vi "MOKE_meas.vi"() -> ()   [LabVIEW 2017]
doc: "Use this template to build a producer/consumer design pattern with events to produce queue items. Use this design pattern instead of the User Interface Event Handler pattern for user interfaces when you want to execute code asynchronously in response to an event without slowing the user interface responsiveness."
uses:
  StateMachine.ctl
  Xaxis.ctl
  Yaxis.ctl
  Meas_arrays.ctl
  <vilib>/DAQmx/write.llb/DAQmx Write (Analog DBL 1Chan 1Samp).vi
  <vilib>/DAQmx/read.llb/DAQmx Read (Analog DBL 1Chan 1Samp).vi
  <vilib>/Analysis/baseanly.llb/Mean (DBL).vi
  <vilib>/DAQmx/read.llb/DAQmx Read (Analog 1D DBL 1Chan NSamp).vi
  <vilib>/DAQmx/read.llb/DAQmx Read (Analog 1D Wfm NChan NSamp).vi
  <vilib>/DAQmx/create/channels.llb/DAQmx Create Channel (AO-Voltage-Basic).vi
  <vilib>/DAQmx/miscellaneous.llb/DAQmx Fill In Error Info.vi
  <vilib>/DAQmx/create/channels.llb/DAQmx Create Channel (AI-Voltage-Basic).vi
  <vilib>/express/express shared/transition.llb/Dynamic To Waveform Array.vi
  <vilib>/express/express arith-compare/Formula/Block/exnFormulaBlock how many pts in the wave.vi
  <vilib>/express/express shared/ex_Modify Signal Name.vi
  <vilib>/express/express shared/transition.llb/Waveform Array To Dynamic.vi
  <vilib>/DAQmx/configure/timing.llb/DAQmx Timing (Sample Clock).vi
  <vilib>/express/express arith-compare/Formula/XNode/ExpressFormulaBlockNode.xnode
  <vilib>/Analysis/NI_AALBase.lvlib
  <vilib>/Analysis/NI_AALPro.lvlib
panel:
  out "Magnetic Bgr":dbl format="%0.2f"
  in  "Plot?":bool=TRUE
  in  "Set Field":bool
  in  "Solenoid Current (A)":dbl
  in  "Magnetization Curve":bool
  in  "Averaging":i32
  in  "Next pt (ms)":u32
  in  "Dwell Time (ms)":u32
  in  "stop 2":bool
  in  "Calibration  (V/deg)":dbl=1.0
  in  "DC normalized?":bool
  out "Array":dbl[](array[numeric])
  out "subarray":dbl[](array[numeric])
  out "LockIn A":dbl[][](array[numeric])
  in  "Current Step (A)":dbl
  in  "Up/dn":bool=TRUE
  in  "Actual Current (A)":dbl
  in  "Max Current (A)":dbl
  in  "Min Current (A)":dbl
  in  "Sweep Field":bool
  in  "Enqueue Element":bool
  in  "Magnet position (mm)":dbl
  in  "Magnet Offset (mm)":dbl=12.5
  in  "Reset":bool
  in  "Continuous":bool
  in  "Polarity":bool
  in  "milliseconds to wait":u32=200
  in  "Tab Control":T1(tab)
  out "Temperature (K)":dbl
  in  "New File":bool
  in  "Measurement File":string
  in  "X axis":T2
  in  "Y axis":T3
  out "Lock-in X, Y":T4(graph)
  in  "X axis 3":T2
  out "MOKE 2":T5(graph)
  in  "Save Data":bool
  out "Magnetic Field (mT)":dbl
  in  "X axis 2":T2
  in  "Y axis 2":T3
  out "dm/dH":T5(graph)
  in  "Delete Calibration":bool
  in  "Measure":bool
  in  "Analyzer angle":dbl step=0.2
  out "MOKE Calibration":cluster{dbl[], "Best Linear Fit":dbl[]}[](graph)
  out "Waveform Graph 2":waveform(dbl)[](graph)
  out "Waveform Graph":waveform(dbl)[](graph)
  in  "DAQ Max voltage":dbl=5.0 format="%0.2f"
  in  "DAQ Min voltage":dbl=-5.0 format="%0.2f"
  in  "DAQ Sample Rate (Hz)":dbl=1000.0
  in  "physical channels":tag="Dev1/ai0:1"
  in  "samples per channel":i32=1000
  in  "Lakeshore VISA":refnum<visa-resource-name>="GPIB0::12::INSTR"
  in  "Keithley or myDAQ":bool=TRUE
  in  "Keithley VISA":refnum<visa-resource-name>="GPIB0::20::INSTR"
  in  "myDAQ":bool
  in  "PT1000 Measure":tag="Dev1/ai1:2"
  in  "minimum value Pt":dbl format="%0.2f"
  in  "maximum value Pt":dbl=5.0 format="%0.2f"
  in  "Dc Intensity PT1000":tag="Dev1/ao1"
  in  "Hall-sensor calibration (mV/mT)":dbl=14.0 format="%0.2f"
  in  "maximum value Hall":dbl=5.0 format="%0.2f"
  in  "minimum value Hall":dbl format="%0.2f"
  in  "Dc Intensity Hall":tag="Dev1/ao0"
  in  "Lockin A, Harmonic":bool=TRUE
  in  "LockIn A VISA":refnum<visa-resource-name>="GPIB0::9::INSTR"
  in  "LockIn B VISA":refnum<visa-resource-name>="GPIB0::9::INSTR"
  in  "Lockin B, Harmonic":bool=TRUE
  in  "Dual Lockin":bool
  in  "Detektor DAQ?":bool
  in  "Hall Measure F":tag="Dev1/ai0"
  in  "Hall Measure":tag="Dev1/ai0"
  in  "Detector signal":tag="Dev1/ai3"
  out "PID signal":dbl
  in  "Goal Temperature (K)":dbl=300.0
  in  "Parameters":cluster{"P":dbl, "I":dbl, "D":dbl}={"P"=1.0, "I"=2.0, "D"=0.0}
  in  "PID On/Off":bool
  in  "Plus Resistance":dbl
  in  "Measurement Arrays":T6
  out "Actual Measurement":T7={"Elapsed Time (s)"=0.0, "Hall-Sensor (mT)"=0.0, "LockIn A"=[1.33515e-05, 1.14442e-05, 1.90736e-05, 41.634], "LockIn B"=[1.33515e-05, 1.14442e-05, 1.90736e-05, 41.634], "Dc Intensity (V)"=0.0, "Temperature (K)"=0.0}
  out "StateMachine":T8
  in  "stop":bool
  # "+"
  # "-"
  # "1f"
  # "2f"
  # "1f"
  # "2f"
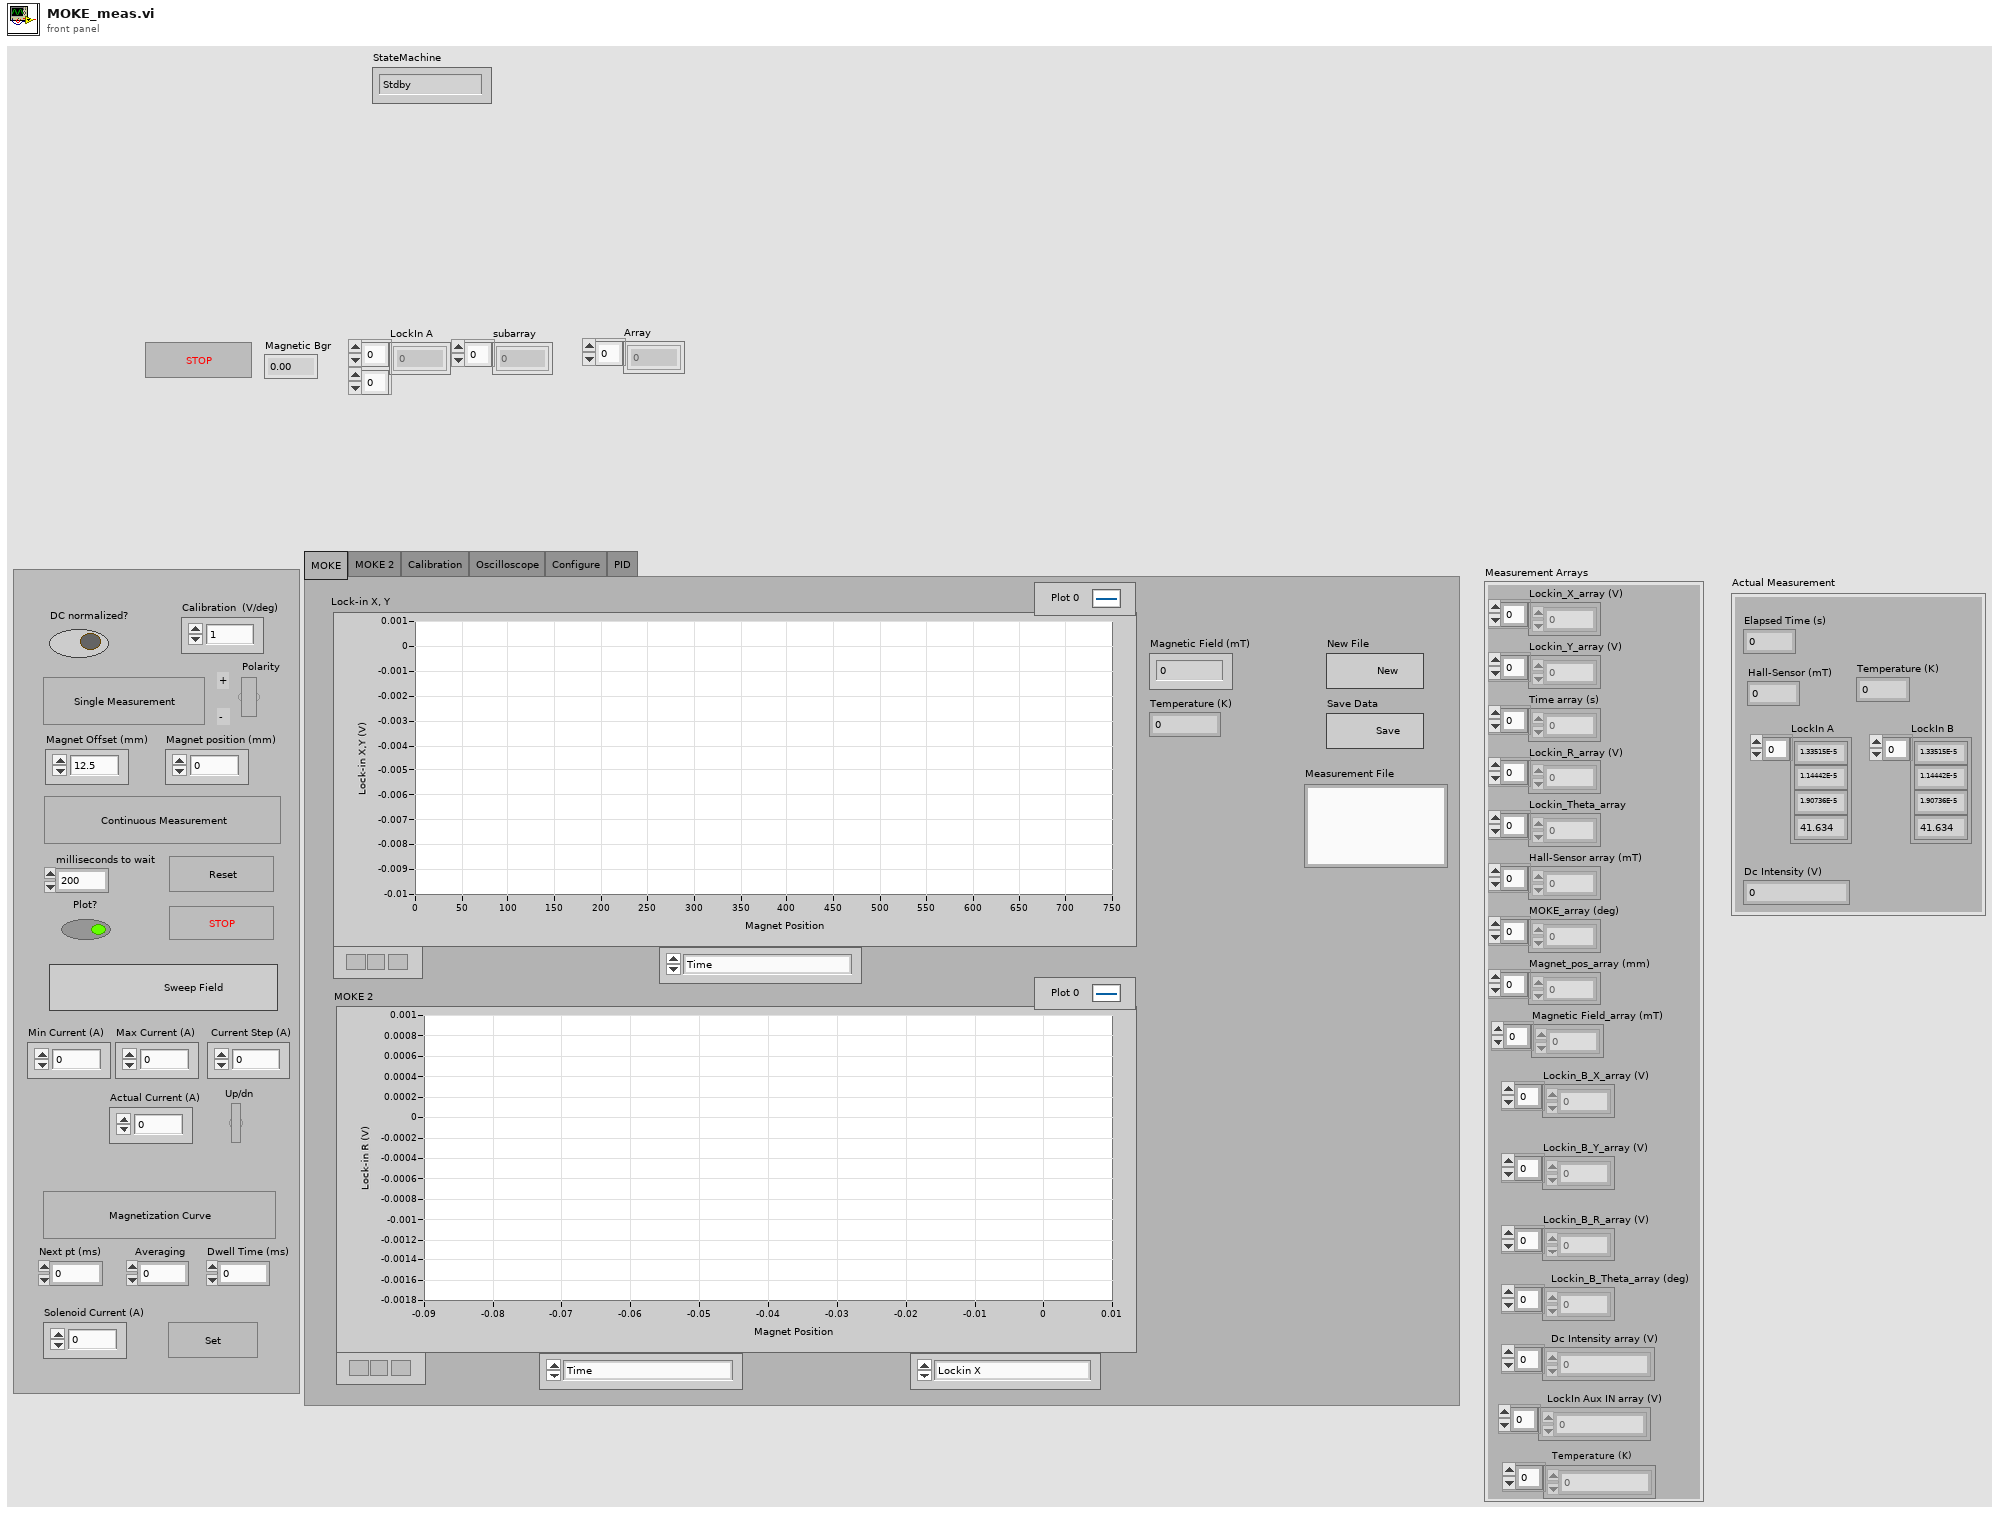
[diagram p1: front panel]
types:
  T1 = enum32{"MOKE", "MOKE 2", "Calibration", "Oscilloscope", "Configure", "PID"}
  T2 = typedef "Xaxis.ctl" = enum16{"Time", "Magnetic Field", "Magnet Position", "Hall Sensor"}
  T3 = typedef "Yaxis.ctl" = enum16{"Lockin X", "Lockin Y", "Lockin R", "Lockin Theta", "MOKE (deg)", "Dc Intensity (V)"}
  T4 = cluster{"Hall-voltage array (V)":dbl[], "Lockin_Y_array (V)":dbl[]}[]
  T5 = cluster{"Magnet_pos_array (mm)":dbl[], "Dc_Voltage_array (V)":dbl[]}
  T6 = typedef "Meas_arrays.ctl" = cluster{"Lockin_X_array (V)":dbl[], "Lockin_Y_array (V)":dbl[], "Time array (s)":dbl[], "Lockin_R_array (V)":dbl[], "Lockin_Theta_array":dbl[], "Hall-Sensor array (mT)":dbl[], "MOKE_array (deg)":dbl[], "Magnet_pos_array (mm)":dbl[], "Magnetic Field_array (mT)":dbl[], "Lockin_B_X_array (V)":dbl[], "Lockin_B_Y_array (V)":dbl[], "Lockin_B_R_array (V)":dbl[], "Lockin_B_Theta_array (deg)":dbl[], "Dc Intensity array (V)":dbl[], "LockIn Aux IN array (V)":dbl[], "Temperature (K)":dbl[]}
  T7 = cluster{"Elapsed Time (s)":dbl, "Hall-Sensor (mT)":dbl, "LockIn A":dbl[], "LockIn B":dbl[], "Dc Intensity (V)":dbl, "Temperature (K)":dbl}
  T8 = typedef "StateMachine.ctl" = enum16{"Stdby", "Configure", "Acquire", "Continuous", "Oscilloscope", "Magnetization", "Calibrate", "PID"}
  T9 = cluster{"Elapsed Time (s)":dbl, "Hall-sensor (mT)":dbl, "LockIn A":dbl[], "LockIn B":dbl[], "Dc Intensity (V)":dbl, "Temperature (K)":dbl}
  T10 = cluster{"Hall-voltage array (V)":dbl[], "Dc Intensity array (V)":dbl[]}
  T11 = cluster{"Hall-voltage array (V)":dbl[], "MOKE_array (deg)":dbl[]}
  T12 = enum16{"open", "replace", "create", "open or create", "replace or create", "replace or create with confirmation"}
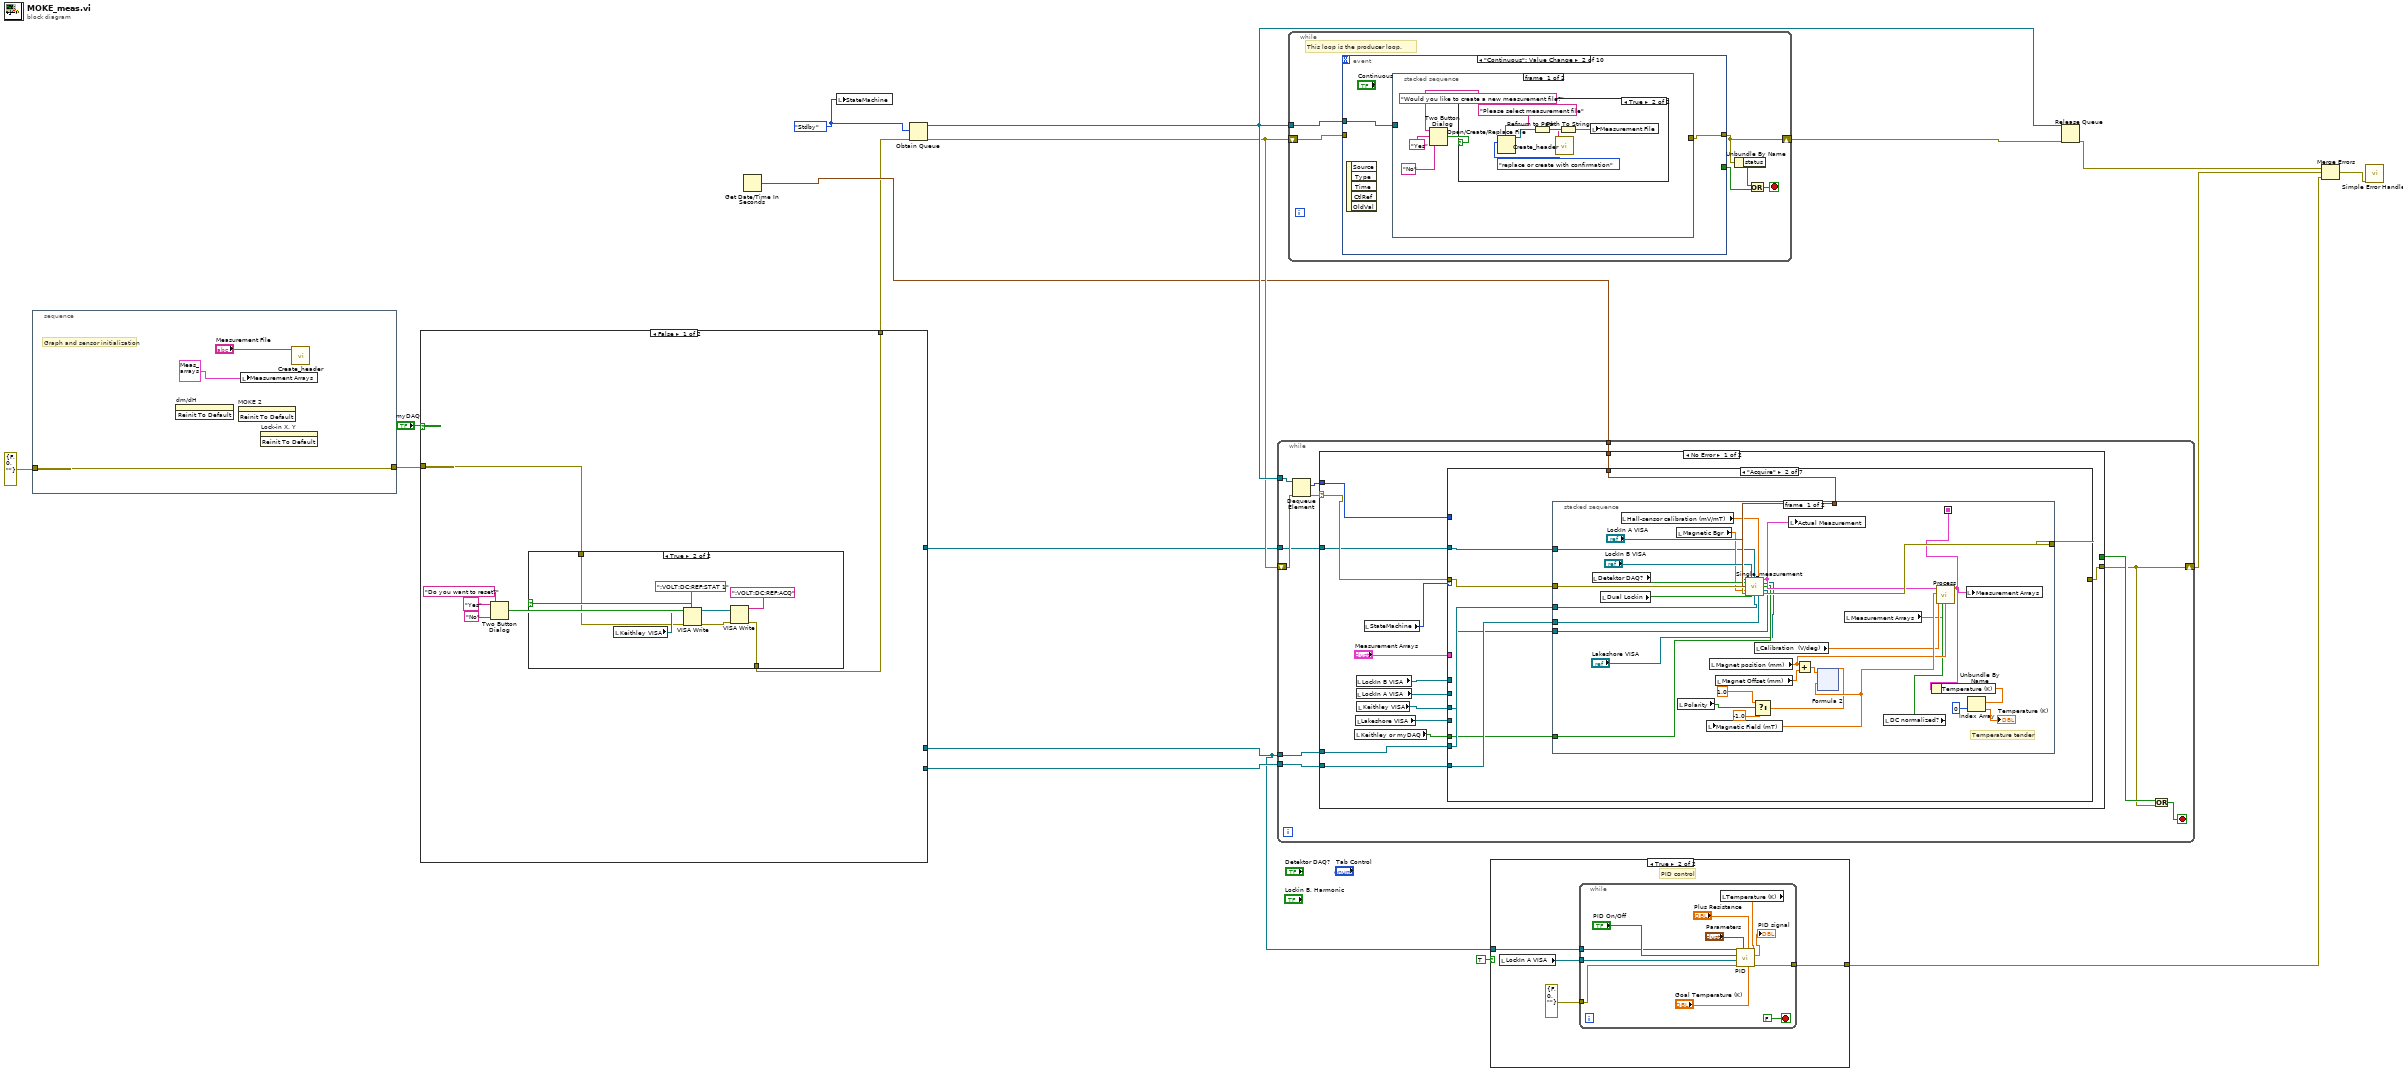
[diagram p0: block diagram]
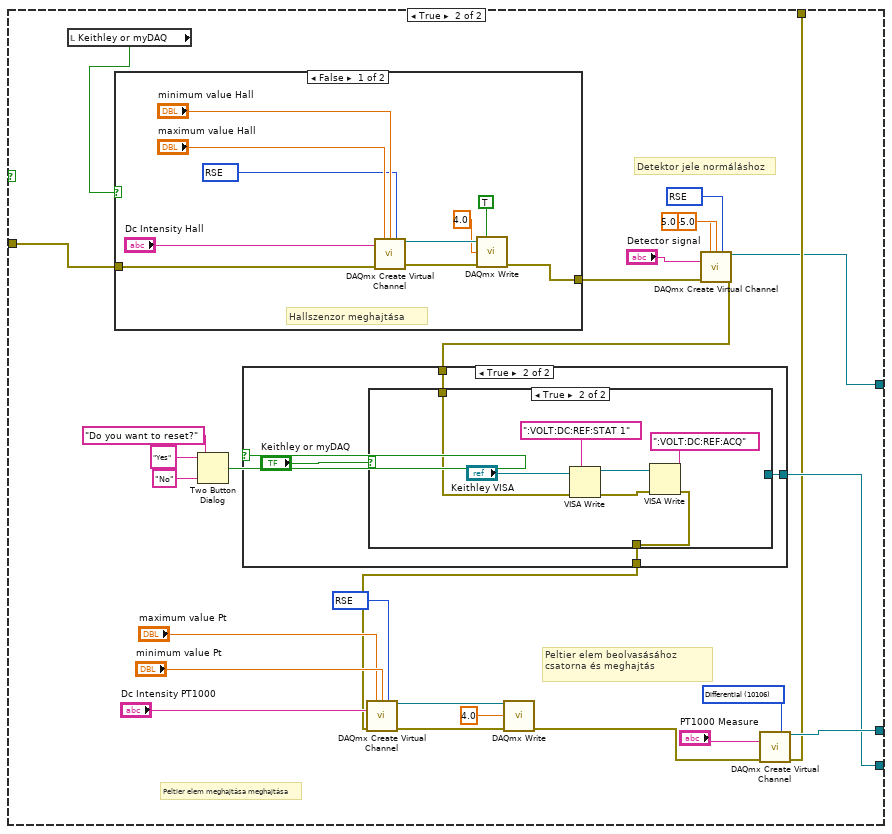
[diagram p4: hidden frame]
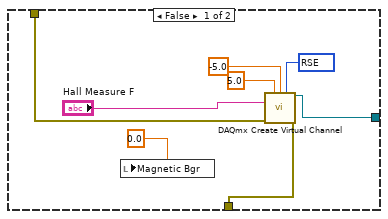
[diagram p6: hidden frame]
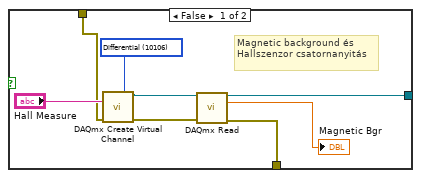
[diagram p7: hidden frame]
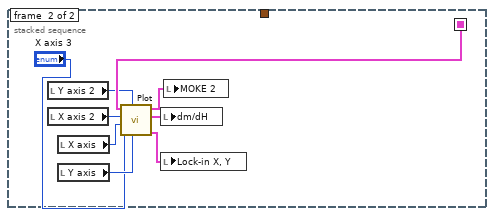
[diagram p9: hidden frame]
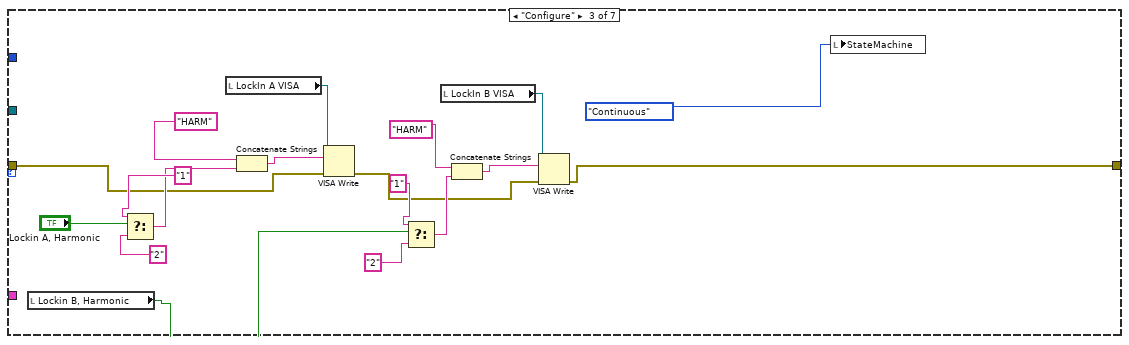
[diagram p10: hidden frame]
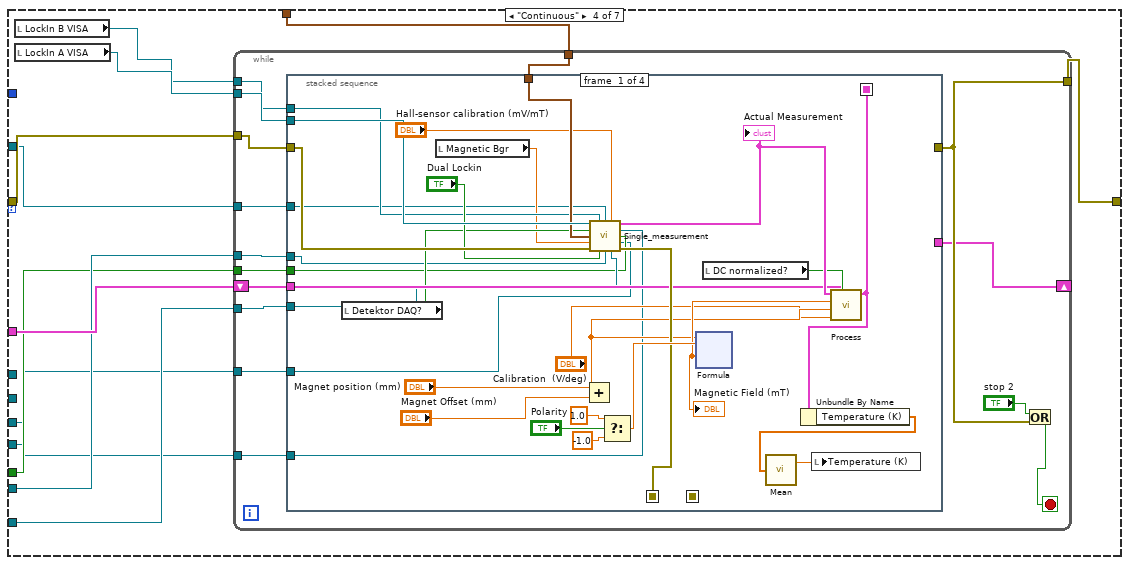
[diagram p11: hidden frame]
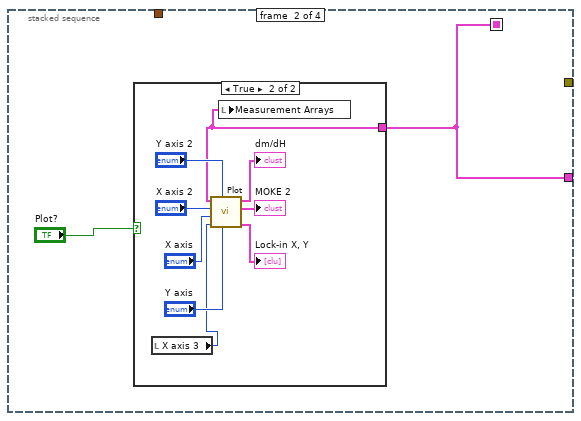
[diagram p12: hidden frame]
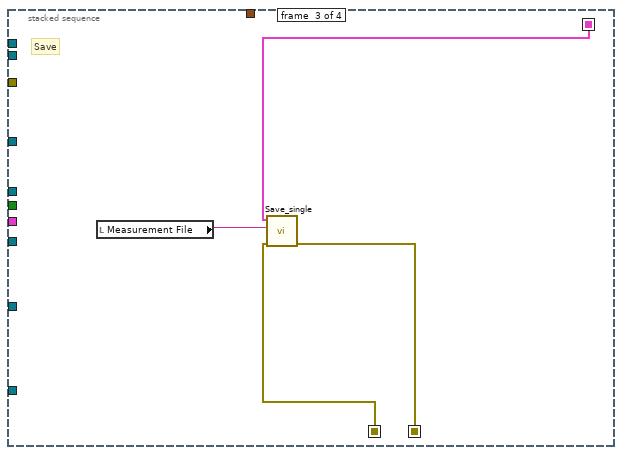
[diagram p14: hidden frame]
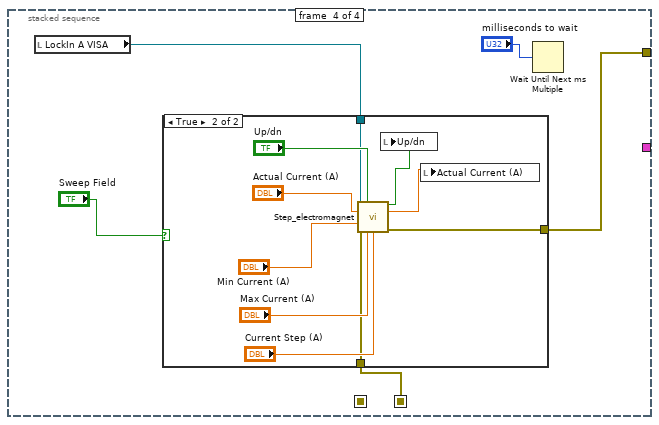
[diagram p15: hidden frame]
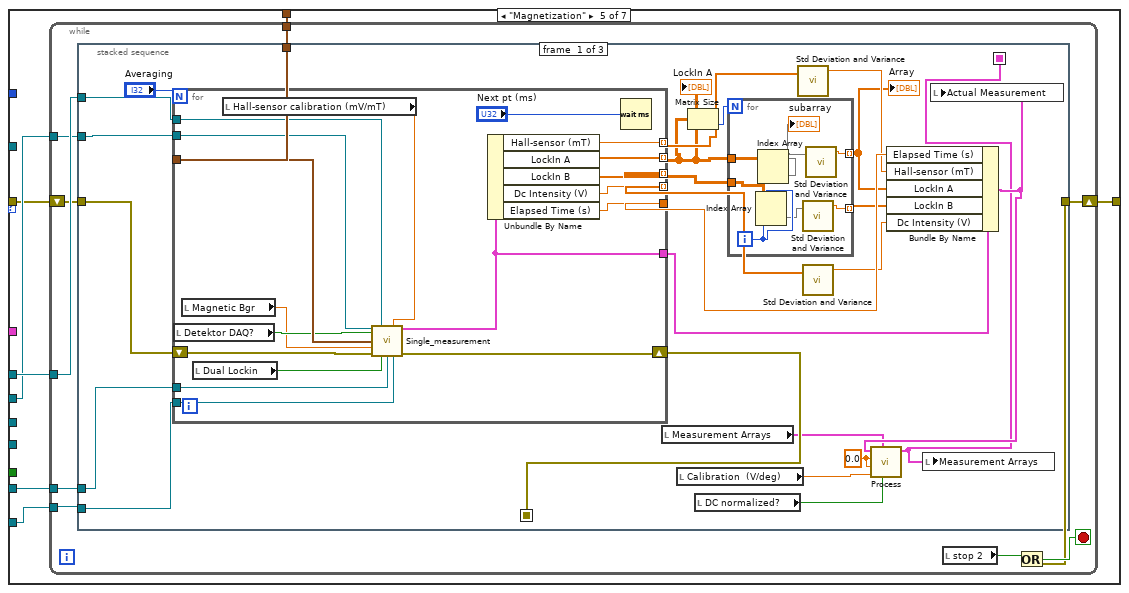
[diagram p17: hidden frame]
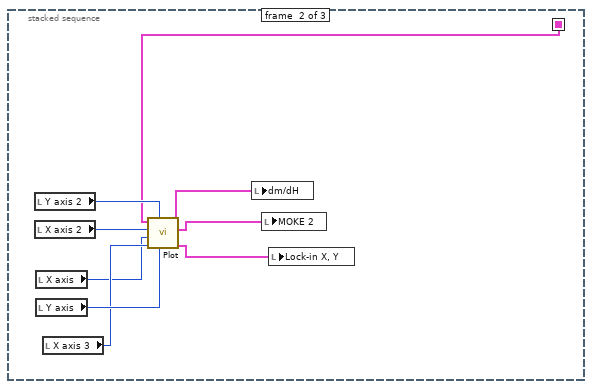
[diagram p18: hidden frame]
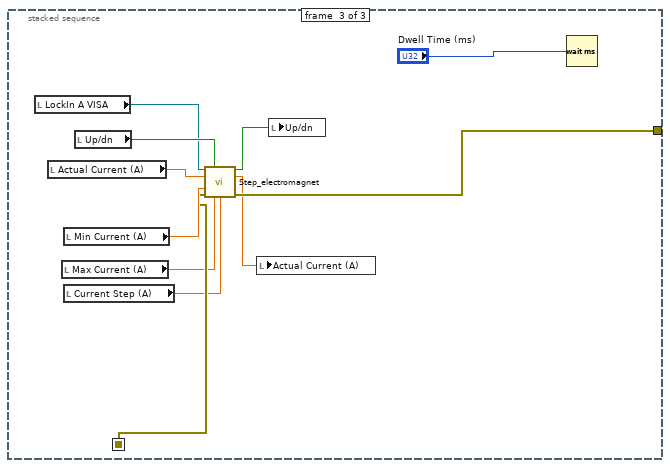
[diagram p19: hidden frame]
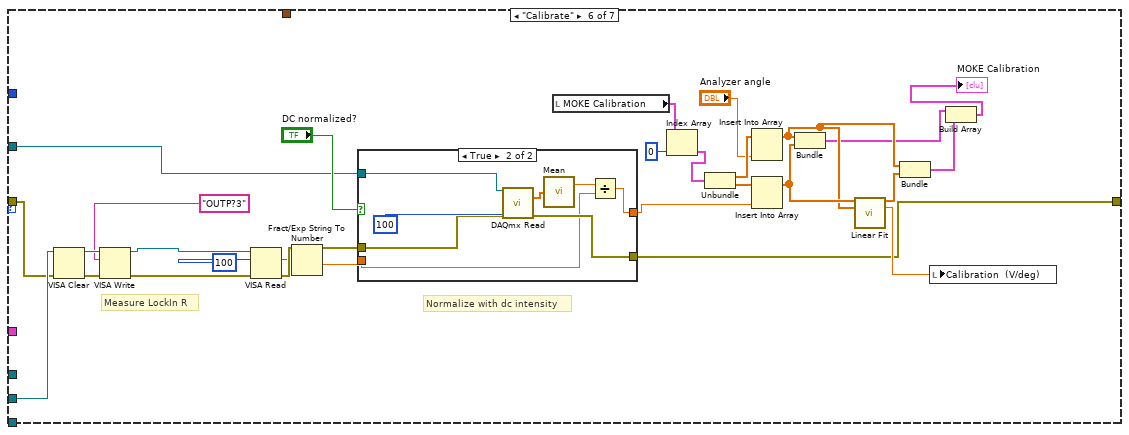
[diagram p20: hidden frame]
diagram:
  w13 = StateMachine."Stdby" ("Enum")
  n1 = stacked-sequence {
    tunnel: errorcluster {"status"=FALSE, "code"=0, "source"=""} ("error out") -> [w20]
    tunnel: [w20] -> w8
    frame #0 {
      # "Graph and sensor initialization"
      n2 = invoke on="dm/dH" class="XYGraph (strict)" method="Reinit To Default"() -> ()  [unwired: 3 in, 3 out]
      n3 = invoke on="MOKE 2" class="XYGraph (strict)" method="Reinit To Default"() -> ()  [unwired: 3 in, 3 out]
      n4 = local write "Measurement Arrays"(T6 {"Lockin_X_array (V)"=[], "Lockin_Y_array (V)"=[], "Time array (s)"=[], "Lockin_R_array (V)"=[], "Lockin_Theta_array"=[], "Hall-Sensor array (mT)"=[], "MOKE_array (deg)"=[], "Magnet_pos_array (mm)"=[], "Magnetic Field_array (mT)"=[], "Lockin_B_X_array (V)"=[], "Lockin_B_Y_array (V)"=[], "Lockin_B_R_array (V)"=[], "Lockin_B_Theta_array (deg)"=[], "Dc Intensity array (V)"=[], "LockIn Aux IN array (V)"=[], "Temperature (K)"=[]} ("Measurement Arrays")) -> ()
      n5 = invoke on="Lock-in X, Y" class="XYGraph (strict)" method="Reinit To Default"() -> ()  [unwired: 3 in, 3 out]
      n6 = call "Create_header.vi"("Measurement File"="Measurement File") -> ()  [unwired: 11 in]
    }
  }
  n7 = case shown="False" "myDAQ" {
    tunnel: [w21 w49] -> w12
    tunnel: w8 -> [w22 w58]
    tunnel: [_ w51] -> w3
    tunnel: [_ w50] -> w6
    tunnel: [_ w45] -> w5
    frame False {
      n8 = Two Button Dialog(message="Do you want to reset?", 1:"No" ("F button name (\"Cancel\")"), 2:"Yes" ("T button name (\"OK\")")) -> (T button?=w23:bool)
      n9 = case shown="True" w23 {
        tunnel: [w27 w28] -> w21
        tunnel: w22 -> [w27 w29]
        frame False {
        }
        frame True {
          n10 = local read "Keithley VISA"() -> (w32:refnum<visa-resource-name>)
          n11 = VISA Write(VISA resource name=w32, write buffer=":VOLT:DC:REF:STAT 1", error in (no error)=w29) -> (VISA resource name out=w33:refnum<visa-resource-name>, error out=w34:errorcluster)  [unwired: 1 out]
          n12 = VISA Write(VISA resource name=w33, write buffer=":VOLT:DC:REF:ACQ", error in (no error)=w34) -> (error out=w28:errorcluster)  [unwired: 2 out]
        }
      }
    }
    frame True {
      w38 = 10083 items=["Default"=-1, "RSE"=10083, "Differential"=10106, "Pseudodifferential"=12529] ("output terminal configuration")
      w39 = 10106 items=["Default"=-1, "RSE"=10083, "NRSE"=10078, "Differential"=10106, "Pseudodifferential"=12529] ("input terminal configuration")
      w42 = 10083 items=["Default"=-1, "RSE"=10083, "NRSE"=10078, "Differential"=10106, "Pseudodifferential"=12529] ("input terminal configuration")
      # "Detektor jele normáláshoz"
      # "Peltier elem beolvasásához csatorna és meghajtás"
      # "Peltier elem meghajtása meghajtása"
      n13 = local read "Keithley or myDAQ"() -> (w35:bool)
      n14 = case shown="False" w35 {
        tunnel: w58 -> [w68 w72]
        tunnel: [w62 w72] -> w36
        frame False {
          w69 = 10083 items=["default"=-1, "RSE"=10083, "NRSE"=10078, "Differential"=10106, "Pseudodifferential"=12529] ("input terminal configuration")
          # "Hallszenzor meghajtása"
          n15 = call-poly <vilib>:"DAQmx Create Virtual Channel.vi"("maximum value"="maximum value Hall", "minimum value"="minimum value Hall", "output terminal configuration"=w69, "physical channels"="Dc Intensity Hall", "error in"=w68) -> ("task out"=w66:refnum<k21>, "error out"=w65:errorcluster)  [unwired: 9 in]
          n16 = call-poly <vilib>:"DAQmx Write.vi"("task/channels in"=w66, "auto start"=TRUE, "data"=4.0, "error in"=w65) -> ("error out"=w62:errorcluster)  [unwired: 9 in, 2 out]
        }
        frame True {
        }
      }
      n17 = Two Button Dialog(message="Do you want to reset?", 1:"No" ("F button name (\"Cancel\")"), 2:"Yes" ("T button name (\"OK\")")) -> (T button?=w54:bool)
      n18 = call-poly <vilib>:"DAQmx Create Virtual Channel.vi"("maximum value"=5.0, "minimum value"=-5.0, "input terminal configuration"=w42, "physical channels"="Detector signal", "error in"=w36) -> ("task out"=w45:refnum<k21>, "error out"=w44:errorcluster)  [unwired: 9 in]
      n19 = case shown="True" w54 {
        tunnel: w44 -> [w77 w84]
        tunnel: [w76 w83] -> w53
        tunnel: [w78 w82] -> w50
        frame False {
          w75 = 10083 items=["Default"=-1, "RSE"=10083, "NRSE"=10078, "Differential"=10106, "Pseudodifferential"=12529] ("input terminal configuration")
          n20 = local write "Magnetic Bgr"(0.0 ("data")) -> ()
          n21 = call-poly <vilib>:"DAQmx Create Virtual Channel.vi"("maximum value"=5.0, "minimum value"=-5.0, "input terminal configuration"=w75, "physical channels"="Hall Measure F", "error in"=w77) -> ("task out"=w78:refnum<k21>, "error out"=w76:errorcluster)  [unwired: 9 in]
        }
        frame True {
          n22 = case shown="True" "Keithley or myDAQ" {
            tunnel: w84 -> [w90 w99]
            tunnel: [w86 w95] -> w83
            tunnel: [w85 _] -> w82
            frame False {
              w87 = 10106 items=["Default"=-1, "RSE"=10083, "NRSE"=10078, "Differential"=10106, "Pseudodifferential"=12529] ("input terminal configuration")
              # "Magnetic background és Hallszenzor csatornanyitás"
              n23 = call-poly <vilib>:"DAQmx Create Virtual Channel.vi"("input terminal configuration"=w87, "physical channels"="Hall Measure", "error in"=w90) -> ("task out"=w88:refnum<k21>, "error out"=w89:errorcluster)  [unwired: 11 in]
              n24 = call-poly <vilib>:"DAQmx Read.vi"("task/channels in"=w88, "error in"=w89) -> ("task out"=w85:refnum<k21>, "data"=→"Magnetic Bgr":dbl, "error out"=w86:errorcluster)  [unwired: 11 in]
            }
            frame True {
              n25 = VISA Write(VISA resource name="Keithley VISA", write buffer=":VOLT:DC:REF:STAT 1", error in (no error)=w99) -> (VISA resource name out=w94:refnum<visa-resource-name>, error out=w96:errorcluster)  [unwired: 1 out]
              n26 = VISA Write(VISA resource name=w94, write buffer=":VOLT:DC:REF:ACQ", error in (no error)=w96) -> (error out=w95:errorcluster)  [unwired: 2 out]
            }
          }
        }
      }
      n27 = call-poly <vilib>:"DAQmx Create Virtual Channel.vi"("maximum value"="maximum value Pt", "minimum value"="minimum value Pt", "output terminal configuration"=w38, "physical channels"="Dc Intensity PT1000", "error in"=w53) -> ("task out"=w48:refnum<k21>, "error out"=w47:errorcluster)  [unwired: 9 in]
      n28 = call-poly <vilib>:"DAQmx Write.vi"("task/channels in"=w48, "data"=4.0, "error in"=w47) -> ("error out"=w37:errorcluster)  [unwired: 10 in, 2 out]
      n29 = call-poly <vilib>:"DAQmx Create Virtual Channel.vi"("input terminal configuration"=w39, "physical channels"="PT1000 Measure", "error in"=w37) -> ("task out"=w51:refnum<k21>, "error out"=w49:errorcluster)  [unwired: 11 in]
    }
  }
  n30 = Get Date/Time In Seconds() -> (seconds since 1Jan1904=w14:timestamp)
  n31 = local write "StateMachine"(w13) -> ()
  n32 = Obtain Queue(element data type=w13, error in (no error)=w12) -> (queue out=w16:refnum<queue>, error out=w15:errorcluster)  [unwired: 3 in, 1 out]
  n33 = while {
    tunnel: w16 -> [w110]
    shift-right: [w104] -> w10
    shift-left: w15 -> [w107]
    tunnel: w14 -> [w106]
    tunnel: w3 -> [w102]
    tunnel: w6 -> [w101]
    tunnel: w5 -> [w100]
    stop <- w103 stop-if-true
    n34 = Dequeue Element(queue=w110, error in (no error)=w107) -> (element=w108:T8, error out=w109:errorcluster)  [unwired: 1 in, 2 out]
    n35 = case shown="No Error" w109 {
      selector: w109 -> [w124 w570]
      tunnel: w108 -> [w122 _]
      tunnel: [_ TRUE] -> w105
      tunnel: [w121 w570] -> w104
      tunnel: w106 -> [w120 _]
      tunnel: w102 -> [w116 _]
      tunnel: w101 -> [w115 _]
      tunnel: w100 -> [w114 _]
      frame No Error {
        n36 = local read "Keithley or myDAQ"() -> (w112:bool)
        n37 = local read "Lakeshore VISA"() -> (w111:refnum<visa-resource-name>)
        n38 = local read "LockIn B VISA"() -> (w119:refnum<visa-resource-name>)
        n39 = local read "LockIn A VISA"() -> (w118:refnum<visa-resource-name>)
        n40 = local read "Keithley VISA"() -> (w113:refnum<visa-resource-name>)
        n41 = local read "StateMachine"() -> (w123:T8)
        n42 = case shown="\"Acquire\"" w123 {
          tunnel: w124 -> [w125 w132 w187 w211 w432 w516 _]
          tunnel: w122 -> [_ _ _ _ _ _ _]
          tunnel: [w125 w131 w185 w210 w431 w517 w556] -> w121
          tunnel: w120 -> [_ w133 _ w212 w433 _ _]
          tunnel: w119 -> [_ _ _ _ w435 _ _]
          tunnel: w118 -> [_ _ _ _ w434 w528 _]
          tunnel: "Measurement Arrays" -> [_ _ _ w208 _ _ _]
          tunnel: w116 -> [_ w130 _ w206 w429 _ _]
          tunnel: w115 -> [_ w129 _ w207 w430 _ _]
          tunnel: w114 -> [_ w128 _ w205 _ w515 _]
          tunnel: w112 -> [_ w127 _ w204 _ _ _]
          tunnel: w113 -> [_ w126 _ w203 _ _ _]
          tunnel: w111 -> [_ _ _ w202 _ _ _]
          frame "Stdby", Default {
          }
          frame "Acquire" {
            n43 = stacked-sequence {
              seq-local: [w144 _] -> [_ w180]
              tunnel: w133 -> [w164 _]
              tunnel: w132 -> [w159 _]
              tunnel: [w158 _] -> w131
              tunnel: w130 -> [w146 _]
              tunnel: w129 -> [w145 _]
              tunnel: w128 -> [w142 _]
              tunnel: w127 -> [w140 _]
              tunnel: w126 -> [w139 _]
              frame #0 {
                # "Temperature tender"
                n44 = local read "Detektor DAQ?"() -> (w147:bool)
                n45 = local read "Dual Lockin"() -> (w148:bool)
                n46 = local read "Hall-sensor calibration (mV/mT)"() -> (w138:dbl)
                n47 = local read "Magnetic Bgr"() -> (w143:dbl)
                n48 = local read "Polarity"() -> (w152:bool)
                n49 = local read "Magnet position (mm)"() -> (w156:dbl)
                n50 = local read "Magnet Offset (mm)"() -> (w163:dbl)
                n51 = call "Single_measurement.vi"("LockIn VISA"="LockIn A VISA", "LockIn VISA 2"="LockIn B VISA", "Detecror signal"=w142, "Hall-sensor calibration (mV/mT)"=w138, "DAQ?"=w147, "Lakeshore VISA"="Lakeshore VISA", "seconds since 1Jan1904"=w164, "Keithly or myDAQ"=w140, "Magnetic Background"=w143, "Keithley VISA 2"=w139, "error in (no error)"=w159, "Dual Lockin"=w148, "Pt1000"=w146, "Hall"=w145) -> ("Measurement"=w154:T9, "error out"=w158:errorcluster)
                n52 = Select(t=1.0, s=w152, f=-1.0) -> (s? t:f=w141:dbl)
                n53 = local read "Calibration  (V/deg)"() -> (w155:dbl)
                n54 = local write "Actual Measurement"(w154) -> ()
                n55 = Add(x=w156, y=w163) -> (x+y=w162:dbl)
                n56 = xnode "Formula 2"("X1"=w162, "sign"=w141) -> ("Result"=w157:dbl)  [unwired: 1 in, 1 out]
                n57 = local write "Magnetic Field (mT)"(w157) -> ()
                n58 = local read "Measurement Arrays"() -> (w149:T6)
                n59 = local read "DC normalized?"() -> (w150:bool)
                n60 = call "Process.vi"("Normalize?"=w150, "Measurement Arrays IN"=w149, "Calibration Constant (1/deg)"=w155, "Magnet position"=w156, "Magnetic Field (mT)"=w157, "Actual Measurement"=w154) -> ("Measurement Arrays OUT"=w144:T6)  [unwired: 3 in]
                n61 = Unbundle By Name(w144) -> ("Temperature (K)"=w136:dbl[])
                n62 = local write "Measurement Arrays"(w144) -> ()
                n63 = Index Array(array=w136, index=0) -> (element=→"Temperature (K)":dbl)
              }
              frame #1 {
                n64 = local read "Y axis 2"() -> (w177:T3)
                n65 = local read "X axis 2"() -> (w178:T2)
                n66 = local read "X axis"() -> (w183:T2)
                n67 = local read "Y axis"() -> (w182:T3)
                n68 = call "Plot.vi"("Y axis"=w182, "Y axis 2"=w177, "X axis 3"="X axis 3", "X axis"=w183, "X axis 2"=w178, "Measurement Arrays"=w180) -> ("MOKE X,Y"=w176:T4, "MOKE 2"=w181:T10, "MOKE"=w179:T11)  [unwired: 3 in]
                n69 = local write "dm/dH"(w181) -> ()
                n70 = local write "Lock-in X, Y"(w176) -> ()
                n71 = local write "MOKE 2"(w179) -> ()
              }
            }
          }
          frame "Configure" {
            n72 = local read "Lockin B, Harmonic"() -> (w184:bool)
            n73 = Select(t="1" ("string"), s="Lockin A, Harmonic", f="2" ("string")) -> (s? t:f=w195:string)
            n74 = local read "LockIn A VISA"() -> (w194:refnum<visa-resource-name>)
            n75 = Concatenate Strings("HARM" ("string"), w195) -> (w200:string)
            n76 = VISA Write(VISA resource name=w194, write buffer=w200, error in (no error)=w187) -> (error out=w186:errorcluster)  [unwired: 2 out]
            n77 = Select(t="1" ("string"), s=w184, f="2" ("string")) -> (s? t:f=w192:string)
            n78 = local read "LockIn B VISA"() -> (w193:refnum<visa-resource-name>)
            n79 = Concatenate Strings("HARM" ("string"), w192) -> (w188:string)
            n80 = VISA Write(VISA resource name=w193, write buffer=w188, error in (no error)=w186) -> (error out=w185:errorcluster)  [unwired: 2 out]
            n81 = local write "StateMachine"(StateMachine."Continuous" ("StateMachine")) -> ()
          }
          frame "Continuous" {
            n82 = local read "LockIn B VISA"() -> (w209:refnum<visa-resource-name>)
            n83 = local read "LockIn A VISA"() -> (w213:refnum<visa-resource-name>)
            n84 = while {
              tunnel: w213 -> [w228]
              tunnel: w212 -> [w227]
              tunnel: w211 -> [w226]
              tunnel: [w222] -> w210
              tunnel: w209 -> [w225]
              tunnel: w206 -> [w224]
              shift-right: [w221] -> _
              shift-left: w208 -> [w220]
              tunnel: w207 -> [w219]
              tunnel: w205 -> [w218]
              tunnel: w204 -> [w216]
              tunnel: w203 -> [w215]
              tunnel: w202 -> [w214]
              stop <- w217 stop-if-true
              n85 = stacked-sequence {
                seq-local: [w233 _ _ _] -> [_ w399 w409 _]
                seq-local: [w247 _ _ _] -> [_ _ w411 _]
                seq-local: [_ _ w410 _] -> [_ _ _ w413]
                tunnel: w228 -> [w258 _ _ _]
                tunnel: w227 -> [w257 _ _ _]
                tunnel: w226 -> [w254 _ _ _]
                tunnel: [_ _ _ w417] -> w222
                tunnel: w225 -> [w248 _ _ _]
                tunnel: w224 -> [w235 _ _ _]
                tunnel: [_ w399 _ _] -> w221
                tunnel: w220 -> [w241 _ _ _]
                tunnel: w219 -> [w236 _ _ _]
                tunnel: w218 -> [w237 _ _ _]
                tunnel: w216 -> [w231 _ _ _]
                tunnel: w215 -> [w230 _ _ _]
                tunnel: w214 -> [w229 _ _ _]
                frame #0 {
                  n86 = local read "Detektor DAQ?"() -> (w239:bool)
                  n87 = local read "Magnetic Bgr"() -> (w238:dbl)
                  n88 = Add(x="Magnet position (mm)", y="Magnet Offset (mm)") -> (x+y=w244:dbl)
                  n89 = call "Single_measurement.vi"("LockIn VISA"=w258, "LockIn VISA 2"=w248, "Detecror signal"=w237, "Hall-sensor calibration (mV/mT)"="Hall-sensor calibration (mV/mT)", "DAQ?"=w239, "Lakeshore VISA"=w229, "seconds since 1Jan1904"=w257, "Keithly or myDAQ"=w231, "Magnetic Background"=w238, "Keithley VISA 2"=w230, "error in (no error)"=w254, "Dual Lockin"="Dual Lockin", "Pt1000"=w235, "Hall"=w236) -> ("Measurement"=w246:T9, "error out"=w247:errorcluster)
                  "Actual Measurement" <- w246
                  n90 = Select(t=1.0, s="Polarity", f=-1.0) -> (s? t:f=w249:dbl)
                  n91 = xnode "Formula"("X1"=w244, "sign"=w249) -> ("Result"=w245:dbl)  [unwired: 1 in, 1 out]
                  "Magnetic Field (mT)" <- w245
                  n92 = local read "DC normalized?"() -> (w242:bool)
                  n93 = call "Process.vi"("Normalize?"=w242, "Measurement Arrays IN"=w241, "Calibration Constant (1/deg)"="Calibration  (V/deg)", "Magnet position"=w244, "Magnetic Field (mT)"=w245, "Actual Measurement"=w246) -> ("Measurement Arrays OUT"=w233:T6)  [unwired: 3 in]
                  n94 = Unbundle By Name(w233) -> ("Temperature (K)"=w234:dbl[])
                  n95 = call-poly <vilib>:"Mean.vi"("X"=w234) -> ("mean"=w232:dbl)  [unwired: 1 out]
                  n96 = local write "Temperature (K)"(w232) -> ()
                }
                frame #1 {
                  n97 = case shown="True" "Plot?" {
                    tunnel: w399 -> [_ w400]
                    frame False {
                    }
                    frame True {
                      n98 = local read "X axis 3"() -> (w401:T2)
                      n99 = call "Plot.vi"("Y axis"="Y axis", "Y axis 2"="Y axis 2", "X axis 3"=w401, "X axis"="X axis", "X axis 2"="X axis 2", "Measurement Arrays"=w400) -> ("MOKE X,Y"=→"Lock-in X, Y":T4, "MOKE 2"=→"MOKE 2":T10, "MOKE"=→"dm/dH":T11)  [unwired: 3 in]
                      n100 = local write "Measurement Arrays"(w400) -> ()
                    }
                  }
                }
                frame #2 {
                  # "Save"
                  n101 = local read "Measurement File"() -> (w412:string)
                  n102 = call "Save_single.vi"("error in (no error)"=w411, "Measurement File"=w412, "Measurement Arrays"=w409) -> ("error out"=w410:errorcluster)  [unwired: 8 in]
                }
                frame #3 {
                  n103 = local read "LockIn A VISA"() -> (w416:refnum<visa-resource-name>)
                  n104 = case shown="True" "Sweep Field" {
                    tunnel: w413 -> [w418 w424]
                    tunnel: [w418 w423] -> w417
                    tunnel: w416 -> [_ w420]
                    frame False {
                    }
                    frame True {
                      n105 = call "Step_electromagnet.vi"("VISA Refnum in"=w420, "Up/dn in"="Up/dn", "Actual Voltage (V)"="Actual Current (A)", "Min Voltage (V) in"="Min Current (A)", "error in (no error)"=w424, "Max Voltage (V)"="Max Current (A)", "Voltage Step (V)"="Current Step (A)") -> ("Up/dn out"=w419:bool, "Min Voltage (V) out"=w421:dbl, "error out"=w423:errorcluster)  [unwired: 6 in]
                      n106 = local write "Up/dn"(w419) -> ()
                      n107 = local write "Actual Current (A)"(w421) -> ()
                    }
                  }
                  n108 = Wait Until Next ms Multiple(millisecond multiple="milliseconds to wait") -> ()  [unwired: 1 out]
                }
              }
              n109 = Or(x="stop 2", y=w222) -> (x .or. y?=w217:bool)
            }
          }
          frame "Magnetization" {
            n110 = while {
              tunnel: w435 -> [w444]
              tunnel: w434 -> [w443]
              tunnel: w433 -> [w442]
              tunnel: w430 -> [w440]
              shift-right: [w437] -> w431
              shift-left: w432 -> [w441]
              tunnel: w429 -> [w436]
              stop <- w438 stop-if-true
              n111 = stacked-sequence {
                seq-local: [w465 _ _] -> [_ _ w509]
                seq-local: [w451 _ _] -> [_ w495 _]
                tunnel: w444 -> [w468 _ _]
                tunnel: w443 -> [w469 _ _]
                tunnel: w442 -> [w467 _ _]
                tunnel: w441 -> [w466 _ _]
                tunnel: w440 -> [w464 _ _]
                tunnel: [_ _ w506] -> w437
                tunnel: w436 -> [w445 _ _]
                frame #0 {
                  w453 = 0.0 ("Magnetic Field (mT)")
                  n112 = for {
                    N: "Averaging" -> [_]
                    tunnel: w469 -> [w494]
                    tunnel: w468 -> [w493]
                    tunnel: w467 -> [w492]
                    shift-right: [w490] -> w465
                    shift-left: w466 -> [w491]
                    tunnel: w464 -> [w488]
                    tunnel: [w486] -> w458
                    tunnel: [w485] -> w462 mode=indexing
                    tunnel: [w484] -> w449 mode=indexing
                    tunnel: [w483] -> w461 mode=indexing
                    tunnel: [w482] -> w460 mode=indexing
                    tunnel: [w481] -> w459
                    tunnel: w445 -> [w478]
                    n113 = local read "Detektor DAQ?"() -> (w480:bool)
                    n114 = local read "Magnetic Bgr"() -> (w477:dbl)
                    n115 = local read "Dual Lockin"() -> (w489:bool)
                    n116 = local read "Hall-sensor calibration (mV/mT)"() -> (w479:dbl)
                    n117 = call "Single_measurement.vi"("LockIn VISA"=w494, "LockIn VISA 2"=w493, "Hall-sensor calibration (mV/mT)"=w479, "DAQ?"=w480, "seconds since 1Jan1904"=w492, "Magnetic Background"=w477, "error in (no error)"=w491, "Dual Lockin"=w489, "Pt1000"=w478, "Hall"=w488) -> ("Measurement"=w481:T9, "error out"=w490:errorcluster)  [unwired: 4 in]
                    n118 = Unbundle By Name(w481) -> ("Hall-sensor (mT)"=w485:dbl, "LockIn A"=w484:dbl[], "LockIn B"=w483:dbl[], "Dc Intensity (V)"=w482:dbl, "Elapsed Time (s)"=w486:dbl)
                    n119 = Wait (ms)(milliseconds to wait="Next pt (ms)") -> ()  [unwired: 1 out]
                  }
                  "LockIn A" <- w449
                  n120 = local read "Measurement Arrays"() -> (w446:T6)
                  n121 = local read "Calibration  (V/deg)"() -> (w454:dbl)
                  n122 = Matrix Size(0:w449) -> (2:w448:i32)  [unwired: 1 out]
                  n123 = local read "DC normalized?"() -> (w447:bool)
                  n124 = for {
                    N: w448 -> [_]
                    tunnel: w449 -> [w474]
                    tunnel: w461 -> [w473]
                    tunnel: [w476] -> w450 mode=indexing
                    tunnel: [w475] -> w456 mode=indexing
                    i -> [w472]
                    n125 = Index Array(array=w473, index (col)=w472) -> (element=w471:dbl[])  [unwired: 1 in]
                    n126 = Index Array(array=w474, index (col)=w472) -> (element=w470:dbl[])  [unwired: 1 in]
                    "subarray" <- w470
                    n127 = call <vilib>:"Std Deviation and Variance.vi"("X"=w471) -> ("mean"=w475:dbl)  [unwired: 1 in, 2 out]
                    n128 = call <vilib>:"Std Deviation and Variance.vi"("X"=w470) -> ("mean"=w476:dbl)  [unwired: 1 in, 2 out]
                  }
                  "Array" <- w450
                  n129 = call <vilib>:"Std Deviation and Variance.vi"("X"=w462) -> ("mean"=w457:dbl)  [unwired: 1 in, 2 out]
                  n130 = call <vilib>:"Std Deviation and Variance.vi"("X"=w460) -> ("mean"=w455:dbl)  [unwired: 1 in, 2 out]
                  n131 = Bundle By Name(cluster=w459, "Elapsed Time (s)"=w458, "Hall-sensor (mT)"=w457, "LockIn A"=w450, "LockIn B"=w456, "Dc Intensity (V)"=w455) -> (w452:T9)
                  n132 = call "Process.vi"("Normalize?"=w447, "Measurement Arrays IN"=w446, "Calibration Constant (1/deg)"=w454, "Magnet position"=w453, "Magnetic Field (mT)"=w453, "Actual Measurement"=w452) -> ("Measurement Arrays OUT"=w451:T6)  [unwired: 3 in]
                  n133 = local write "Measurement Arrays"(w451) -> ()
                  n134 = local write "Actual Measurement"(w452) -> ()
                }
                frame #1 {
                  n135 = local read "Y axis 2"() -> (w497:T3)
                  n136 = local read "X axis 2"() -> (w496:T2)
                  n137 = local read "X axis"() -> (w498:T2)
                  n138 = local read "Y axis"() -> (w500:T3)
                  n139 = local read "X axis 3"() -> (w499:T2)
                  n140 = call "Plot.vi"("Y axis"=w500, "Y axis 2"=w497, "X axis 3"=w499, "X axis"=w498, "X axis 2"=w496, "Measurement Arrays"=w495) -> ("MOKE X,Y"=w501:T4, "MOKE 2"=w502:T10, "MOKE"=w503:T11)  [unwired: 3 in]
                  n141 = local write "dm/dH"(w503) -> ()
                  n142 = local write "MOKE 2"(w502) -> ()
                  n143 = local write "Lock-in X, Y"(w501) -> ()
                }
                frame #2 {
                  n144 = local read "LockIn A VISA"() -> (w512:refnum<visa-resource-name>)
                  n145 = local read "Actual Current (A)"() -> (w511:dbl)
                  n146 = local read "Max Current (A)"() -> (w508:dbl)
                  n147 = local read "Min Current (A)"() -> (w510:dbl)
                  n148 = local read "Current Step (A)"() -> (w507:dbl)
                  n149 = local read "Up/dn"() -> (w514:bool)
                  n150 = call "Step_electromagnet.vi"("VISA Refnum in"=w512, "Up/dn in"=w514, "Actual Voltage (V)"=w511, "Min Voltage (V) in"=w510, "error in (no error)"=w509, "Max Voltage (V)"=w508, "Voltage Step (V)"=w507) -> ("Up/dn out"=w513:bool, "Min Voltage (V) out"=w505:dbl, "error out"=w506:errorcluster)  [unwired: 6 in]
                  n151 = local write "Actual Current (A)"(w505) -> ()
                  n152 = local write "Up/dn"(w513) -> ()
                  n153 = Wait (ms)(milliseconds to wait="Dwell Time (ms)") -> ()  [unwired: 1 out]
                }
              }
              n154 = local read "stop 2"() -> (w439:bool)
              n155 = Or(x=w439, y=w437) -> (x .or. y?=w438:bool)
            }
          }
          frame "Calibrate" {
            # "Normalize with dc intensity"
            # "Measure LockIn R"
            n156 = VISA Clear(VISA resource name=w528, error in (no error)=w516) -> (VISA resource name out=w541:refnum<visa-resource-name>, error out=w540:errorcluster)
            n157 = VISA Write(VISA resource name=w541, write buffer="OUTP?3" ("data"), error in (no error)=w540) -> (VISA resource name out=w536:refnum<visa-resource-name>, error out=w538:errorcluster)  [unwired: 1 out]
            n158 = VISA Read(VISA resource name=w536, byte count=100, error in (no error)=w538) -> (read buffer=w534:string, error out=w535:errorcluster)  [unwired: 2 out]
            n159 = Fract/Exp String To Number(string=w534) -> (number=w533:dbl)  [unwired: 3 in, 1 out]
            n160 = case shown="True" "DC normalized?" {
              tunnel: w515 -> [_ w551]
              tunnel: w535 -> [w544 w550]
              tunnel: [w544 w549] -> w517
              tunnel: w533 -> [w543 w546]
              tunnel: [w543 w545] -> w529
              frame False {
              }
              frame True {
                n161 = call-poly <vilib>:"DAQmx Read.vi"("task/channels in"=w551, "number of samples per channel"=100, "error in"=w550) -> ("data"=w548:dbl[], "error out"=w549:errorcluster)  [unwired: 10 in, 1 out]
                n162 = call-poly <vilib>:"Mean.vi"("X"=w548) -> ("mean"=w547:dbl)  [unwired: 1 out]
                n163 = Divide(x=w547, y=w546) -> (x/y=w545:dbl)
              }
            }
            n164 = local read "MOKE Calibration"() -> (w521:cluster{dbl[], "Best Linear Fit":dbl[]}[])
            n165 = Index Array(array=w521, index=0) -> (element=w520:cluster{dbl[], "Best Linear Fit":dbl[]})
            n166 = Unbundle(w520) -> (w532:dbl[], "Best Linear Fit"=w530:dbl[])
            n167 = Insert Into Array(array=w532, new element="Analyzer angle") -> (w526:dbl[])  [unwired: 1 in]
            n168 = Insert Into Array(array=w530, new element=w529) -> (w527:dbl[])  [unwired: 1 in]
            n169 = Bundle(w526, "Best Linear Fit"=w527) -> (w524:cluster{dbl[], "Best Linear Fit":dbl[]})  [unwired: 1 in]
            n170 = call <vilib>:"Linear Fit.vi"("Y"=w527, "X"=w526) -> ("Best Linear Fit"=w525:dbl[], "slope"=w518:dbl)  [unwired: 9 in, 3 out]
            n171 = Bundle(w526, "Best Linear Fit"=w525) -> (w523:cluster{dbl[], "Best Linear Fit":dbl[]})  [unwired: 1 in]
            n172 = local write "Calibration  (V/deg)"(w518) -> ()
            n173 = Build Array(w524, w523) -> (→"MOKE Calibration":cluster{dbl[], "Best Linear Fit":dbl[]}[])
          }
          frame "Oscilloscope" {
            w562 = 10106 items=["default"=-1, "RSE"=10083, "NRSE"=10078, "Differential"=10106, "Pseudodifferential"=12529] ("input terminal configuration")
            w565 = 10178 items=["Finite Samples"=10178, "Continuous Samples"=10123, "Hardware Timed Single Point"=12522] ("sample mode")
            n174 = call-poly <vilib>:"DAQmx Create Virtual Channel.vi"("maximum value"="DAQ Max voltage", "minimum value"="DAQ Min voltage", "input terminal configuration"=w562, "physical channels"="physical channels") -> ("task out"=w568:refnum<k21>, "error out"=w567:errorcluster)  [unwired: 10 in]
            n175 = call-poly <vilib>:"DAQmx Timing.vi"("task/channels in"=w568, "sample mode"=w565, "samples per channel"="samples per channel", "rate"="DAQ Sample Rate (Hz)", "error in"=w567) -> ("task out"=w561:refnum<k21>, "error out"=w560:errorcluster)  [unwired: 9 in]
            n176 = call <vilib>:"DAQmx Start Task.vi"("task/channels in"=w561, "error in"=w560) -> ("task out"=w559:refnum<k21>, "error out"=w558:errorcluster)  [unwired: 12 in]
            n177 = call-poly <vilib>:"DAQmx Read.vi"("task/channels in"=w559, "number of samples per channel"="samples per channel", "error in"=w558) -> ("data"=w553:waveform(dbl)[], "error out"=w556:errorcluster)  [unwired: 10 in, 1 out]
            "Waveform Graph" <- w553
            "Waveform Graph 2" <- w553
            n178 = Index Array(array=w553, index=0 ("index (row)")) -> ()  [unwired: 1 out]
            n179 = Index Array(array=w553, index=1 ("index (row)")) -> ()  [unwired: 1 out]
          }
        }
      }
      frame Error {
        # "Return true in any case that should stop the loop."
      }
    }
    n180 = Or(x=w105, y=w104) -> (x .or. y?=w103:bool)
  }
  n181 = while {
    shift-right: [w573] -> w17
    shift-left: w15 -> [w576]
    tunnel: w16 -> [w577]
    stop <- w574 stop-if-true
    # "This loop is the producer loop."
    n182 = event shown="[1] \"Continuous\": Value Change" {
      selector: _ -> [_ _ _ _ _ _ _ _ _ _]
      dyn-events: _ -> [_ _ _ _ _ _ _ _ _ _]
      timeout: _ -> [_ _ _ _ _ _ _ _ _ _]
      tunnel: w577 -> [w580 w582 w598 w599 _ _ _ _ _ _]
      tunnel: w576 -> [_ _ w597 w601 _ _ _ _ w628 w631]
      tunnel: [w579 w581 w596 w600 _ _ _ _ w628 w630] -> w573
      tunnel: [_ _ _ _ _ _ _ _ "stop" _] -> w575
      event "Enqueue Element": Value Change {
        w578 = StateMachine."Acquire" ("Enum")
        n183 = event-data() -> ()  [unwired: 1 in, 1 out]
        n184 = Enqueue Element(queue=w580, element=w578) -> (error out=w579:errorcluster)  [unwired: 2 in, 2 out]
        "StateMachine" <- w578
      }
      event "Continuous": Value Change {
        n185 = event-data() -> ()  [unwired: 1 in, 5 out]
        n186 = stacked-sequence {
          tunnel: w582 -> [_ w594]
          tunnel: [_ w592] -> w581
          frame #0 {
            n187 = Two Button Dialog(message="Would you like to create a new measurement file?", 1:"No" ("F button name (\"Cancel\")"), 2:"Yes" ("T button name (\"OK\")")) -> (T button?=w583:bool)
            n188 = case shown="True" w583 {
              frame False {
              }
              frame True {
                n189 = Open/Create/Replace File(prompt="Please select measurement file", operation (0:open)=T12."replace or create with confirmation") -> (refnum out=w591:refnum<file>)  [unwired: 4 in, 2 out]
                n190 = Refnum to Path(1:w591) -> (0:w590:path)
                n191 = Path To String(path=w590) -> (string=w589:string)
                n192 = call "Create_header.vi"("Measurement File"=w589) -> ()  [unwired: 11 in]
                n193 = local write "Measurement File"(w589) -> ()
              }
            }
          }
          frame #1 {
            w593 = StateMachine."Continuous" ("StateMachine")
            n194 = local write "StateMachine"(w593) -> ()
            n195 = Enqueue Element(queue=w594, element=w593) -> (error out=w592:errorcluster)  [unwired: 2 in, 2 out]
          }
        }
      }
      event "Magnetization Curve": Value Change {
        w595 = StateMachine."Magnetization" ("StateMachine")
        n196 = event-data() -> ()  [unwired: 1 in, 5 out]
        n197 = local write "StateMachine"(w595) -> ()
        n198 = Enqueue Element(queue=w598, element=w595, error in (no error)=w597) -> (error out=w596:errorcluster)  [unwired: 1 in, 2 out]
      }
      event "Measure": Value Change {
        w602 = StateMachine."Calibrate" ("StateMachine")
        n199 = event-data() -> ()  [unwired: 1 in, 5 out]
        n200 = local write "StateMachine"(w602) -> ()
        n201 = Enqueue Element(queue=w599, element=w602, error in (no error)=w601) -> (error out=w600:errorcluster)  [unwired: 1 in, 2 out]
      }
      event "Delete Calibration": Value Change {
        n202 = event-data() -> ()  [unwired: 1 in, 6 out]
        n203 = invoke on="MOKE Calibration" class="XYGraph (strict)" method="Reinit To Default"() -> ()  [unwired: 3 in, 3 out]
      }
      event "Save Data": Value Change {
        n204 = local read "Measurement Arrays"() -> (w604:T6)
        n205 = event-data() -> ()  [unwired: 1 in, 6 out]
        n206 = Unbundle By Name(w604) -> ("Time array (s)"=w616:dbl[], "Magnet_pos_array (mm)"=w619:dbl[], "Magnetic Field_array (mT)"=w618:dbl[], "Hall-Sensor array (mT)"=w617:dbl[], "Lockin_X_array (V)"=w615:dbl[], "Lockin_Y_array (V)"=w614:dbl[], "Lockin_R_array (V)"=w613:dbl[], "Lockin_Theta_array"=w612:dbl[], "LockIn Aux IN array (V)"=w611:dbl[], "MOKE_array (deg)"=w610:dbl[], "Lockin_B_X_array (V)"=w609:dbl[], "Lockin_B_Y_array (V)"=w608:dbl[], "Lockin_B_R_array (V)"=w607:dbl[], "Lockin_B_Theta_array (deg)"=w606:dbl[], "Temperature (K)"=w603:dbl[])
        n207 = Build Array(w616, w619, w618, w617, w615, w614, w613, w612, w611, w610, w609, w608, w607, w606, w603) -> (w605:dbl[][])
        n208 = call "Convert to Dynamic Data"("2D Array"=w605) -> ("Dynamic Data Type"=w620:dynamicdata)  [unwired: 3 in]
        n209 = call "Write To Measurement File"("Signals"=w620) -> ()  [unwired: 16 in, 3 out]
      }
      event "New File": Value Change {
        n210 = event-data() -> ()  [unwired: 1 in, 6 out]
        n211 = Open/Create/Replace File(prompt="Please select measurement file", operation (0:open)=T12."replace or create with confirmation") -> (refnum out=w624:refnum<file>)  [unwired: 4 in, 2 out]
        n212 = Refnum to Path(1:w624) -> (0:w623:path)
        n213 = Path To String(path=w623) -> (string=w621:string)
        n214 = call "Create_header.vi"("Measurement File"=w621) -> ()  [unwired: 11 in]
        n215 = local write "Measurement File"(w621) -> ()
      }
      event "Reset": Value Change {
        (unwired) dbl[] []
        n216 = event-data() -> ()  [unwired: 1 in, 1 out]
        n217 = invoke on="dm/dH" class="XYGraph (strict)" method="Reinit To Default"() -> ()  [unwired: 3 in, 3 out]
        n218 = local write "Measurement Arrays"(T6 {"Lockin_X_array (V)"=[], "Lockin_Y_array (V)"=[], "Time array (s)"=[], "Lockin_R_array (V)"=[], "Lockin_Theta_array"=[], "Hall-Sensor array (mT)"=[], "MOKE_array (deg)"=[], "Magnet_pos_array (mm)"=[], "Magnetic Field_array (mT)"=[], "Lockin_B_X_array (V)"=[], "Lockin_B_Y_array (V)"=[], "Lockin_B_R_array (V)"=[], "Lockin_B_Theta_array (deg)"=[], "Dc Intensity array (V)"=[], "LockIn Aux IN array (V)"=[], "Temperature (K)"=[]} ("Measurement Arrays")) -> ()
      }
      event "stop": Value Change {
        n219 = event-data() -> ()  [unwired: 1 in, 1 out]
        n220 = local write "StateMachine"(StateMachine."Stdby" ("Enum")) -> ()
      }
      event "Set Field": Value Change {
        n221 = event-data() -> ()  [unwired: 1 in, 6 out]
        n222 = Divide(x=5.0 ("y"), y=10.0) -> (x/y=w639:dbl)
        n223 = Multiply(x="Solenoid Current (A)", y=w639) -> (x*y=w636:dbl)
        n224 = Number To Fractional String(number=w636, precision (6)=i16 3) -> (F-format string=w635:string)  [unwired: 2 in]
        n225 = local read "LockIn A VISA"() -> (w633:refnum<visa-resource-name>)
        n226 = Concatenate Strings("AUXV 1," ("data"), w635) -> (w632:string)
        n227 = VISA Write(VISA resource name=w633, write buffer=w632, error in (no error)=w631) -> (error out=w630:errorcluster)  [unwired: 2 out]
      }
    }
    n228 = Unbundle By Name(w573) -> ("status"=w572:bool)
    n229 = Or(x=w572, y=w575) -> (x .or. y?=w574:bool)
  }
  n230 = case shown="True" TRUE {
    tunnel: w3 -> [_ w645]
    tunnel: [_ w644] -> w2
    frame False {
    }
    frame True {
      # "PID control"
      n231 = local read "LockIn A VISA"() -> (w643:refnum<visa-resource-name>)
      n232 = while {
        tunnel: w645 -> [w653]
        tunnel: [w652] -> w644
        tunnel: w643 -> [w650]
        tunnel: errorcluster {"status"=FALSE, "code"=0, "source"=""} ("error in (no error)") -> [w649]
        stop <- FALSE stop-if-true
        n233 = local read "Temperature (K)"() -> (w647:dbl)
        n234 = call "PID.vi"("Refnum in"=w653, "PID On/Off"="PID On/Off", "VISA resource name"=w650, "error in (no error)"=w649, "Parameters"="Parameters", "Plus Resistance"="Plus Resistance", "Goal Temperature (K)"="Goal Temperature (K)", "Temperature"=w647) -> ("PID signal"=→"PID signal":dbl, "error out"=w652:errorcluster)  [unwired: 1 in]
      }
    }
  }
  n235 = Release Queue(queue=w16, error in (no error)=w17) -> (error out=w11:errorcluster)  [unwired: 1 in, 2 out]
  n236 = Merge Errors(w11, w10, w2) -> (w9:errorcluster)
  n237 = call <vilib>:"Simple Error Handler.vi"("error in (no error)"=w9) -> ()  [unwired: 4 in, 5 out]
